vi "DEMO_HOW_TO_USE_CameraManager.vi"() -> ()   [LabVIEW 2017, in "PlayNitrideCameraComponet1010_4.lvlib"]
uses:
  <userlib>/PlayNitrideCameraComponet1010_4/PlayNitrideCameraComponet1010_4.lvlib
panel:
  out "Camera Count":i32
  out "Version":string
  out "Initial Status":bool
  out "Spend Time (ms)":u32
  out "Image":T1(plugin-control)
  in  "Camera Manager Data":T2={"Camera Index"=0.0, "Exposure Time"=2800.0, "Image"=refnum, "Save Img Path"=path "C:/Users/MyUser/Pictures", "error out"={"status"=FALSE, "code"=0, "source"=""}, "Specific Parameter"={"Parameter Name"="", "Parameter Value"=""}, "Image Info"={"Height"=0.0, "Width"=0.0, "Channels"=0.0}}
  out "Camera Manager Data Output":T2={"Camera Index"=0.0, "Exposure Time"=2800.0, "Image"=refnum, "Save Img Path"=path "C:/Users/MyUser/Pictures", "error out"={"status"=FALSE, "code"=0, "source"=""}, "Specific Parameter"={"Parameter Name"="", "Parameter Value"=""}, "Image Info"={"Height"=0.0, "Width"=0.0, "Channels"=0.0}}
  out "Commands In Queue":i32
  out "error out":errorcluster
  out "save img path":path
  in  "Pic Path":path=path "C:/Users/MyUser/Pictures/2-原圖.bmp"
  in  "Cluster In":T3={"Camera Mode"=TRUE, "顯示準星"=FALSE, "準星顏色"=65469}
  in  "Save Setting":T4
  in  "element":cluster{"State":string}
  in  "Select Command":string(combo)
  # "Select Command : 目前可以支援的指令"
  # "Initial Status : 顯示Camera Manager 是否已經成功初始化\nCamera Count: 顯示目前相機數量\n Version: 顯示目前Camera Manager dll 版號 未來用於Debug回報資訊的依據"
  # "Extra Param"
  # "Extra Output"
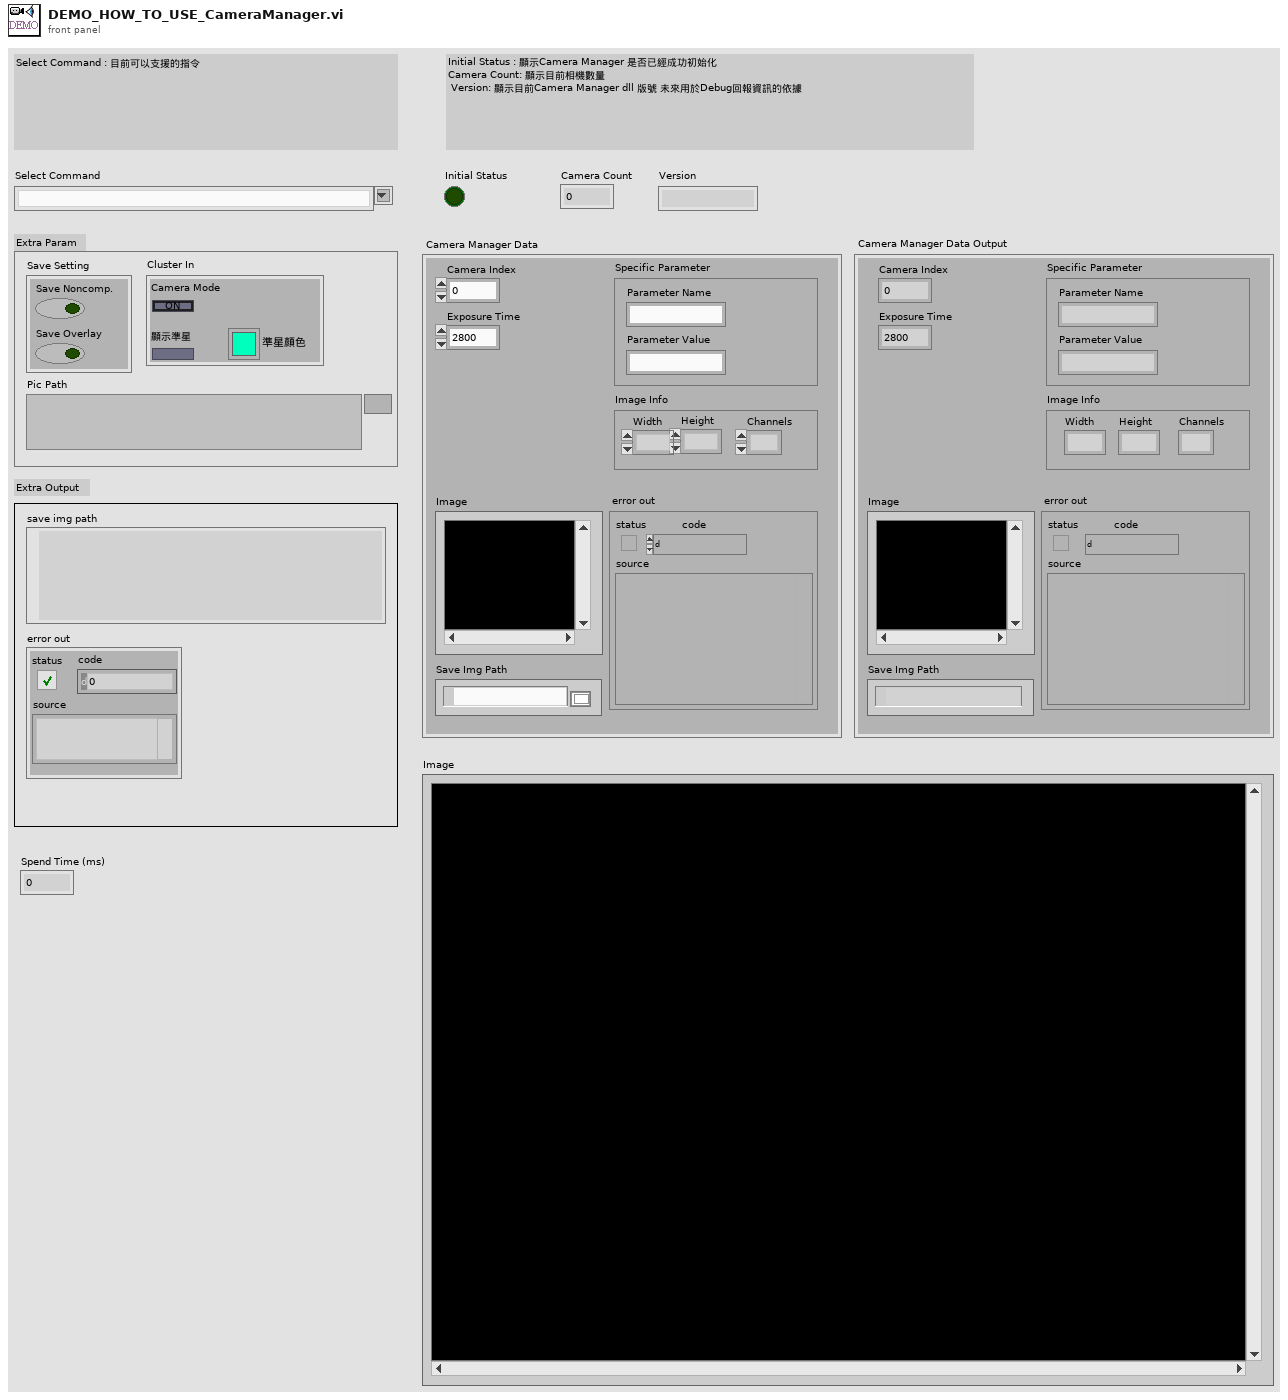
[diagram p1: front panel]
types:
  T1 = typedef "IMAQ Image.ctl" = refnum<image>
  T2 = cluster{"Camera Index":dbl, "Exposure Time":dbl, "Image":T1, "Save Img Path":path, "error out":errorcluster, "Specific Parameter":cluster{"Parameter Name":string, "Parameter Value":string}, "Image Info":cluster{"Height":dbl, "Width":dbl, "Channels":dbl}}
  T3 = cluster{"Camera Mode":bool, "顯示準星":bool, "準星顏色":u32}
  T4 = cluster{"Save Noncomp.":bool, "Save Overlay":bool}
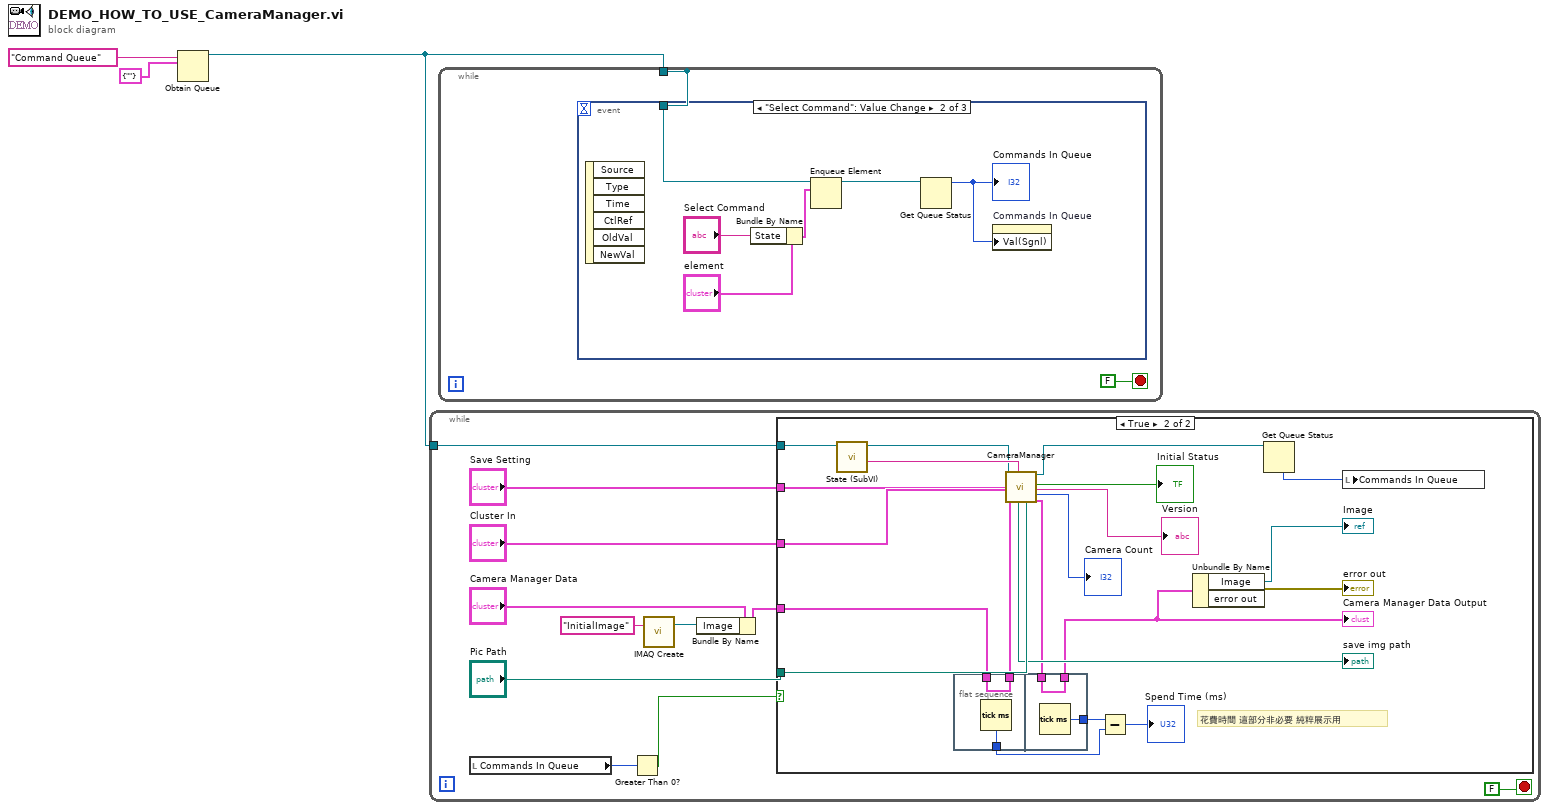
[diagram p0: block diagram]
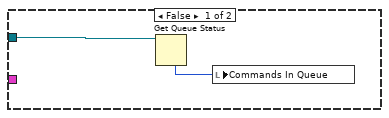
[diagram p2: hidden frame]
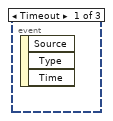
[diagram p3: hidden frame]
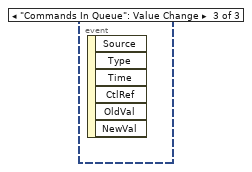
[diagram p4: hidden frame]
diagram:
  n1 = Obtain Queue(name (unnamed)="Command Queue", element data type=cluster{"State":string} {"State"=""}) -> (queue out=w1:refnum<queue>)  [unwired: 3 in, 2 out]
  n2 = while {
    tunnel: w1 -> [w11]
    stop <- FALSE stop-if-true
    n3 = local read "Commands In Queue"() -> (w14:i32)
    n4 = Greater Than 0?(x=w14) -> (x > 0?=w13:bool)
    n5 = call "IMAQ Create"("Image Name"="InitialImage") -> ("New Image"=w4:T1)  [unwired: 4 in, 1 out]
    n6 = Bundle By Name(cluster="Camera Manager Data", "Image"=w4) -> (w6:T2)
    n7 = case shown="True" w13 {
      tunnel: w11 -> [w15 w37]
      tunnel: "Save Setting" -> [_ w29]
      tunnel: "Cluster In" -> [_ w33]
      tunnel: w6 -> [_ w26]
      tunnel: "Pic Path" -> [_ w32]
      frame False {
        n8 = Get Queue Status(queue=w15) -> (# elements in queue=w16:i32)  [unwired: 2 in, 7 out]
        n9 = local write "Commands In Queue"(w16) -> ()
      }
      frame True {
        # "花費時間 這部分非必要 純粹展示用"
        n10 = call <userlib>:"State (SubVI).vi"("Queue in"=w37) -> ("State"=w36:string, "Queue out"=w35:refnum<queue>)  [unwired: 8 in, 1 out]
        n11 = flat-sequence {
          tunnel: [w39] -> w27
          tunnel: w26 -> [w39]
          tunnel: [w38] -> w23
          tunnel: [w41] -> w24
          tunnel: w25 -> [w41]
          tunnel: [w40] -> w22
          frame #0 {
            n12 = Tick Count (ms)() -> (millisecond timer value=w38:u32)
          }
          frame #1 {
            n13 = Tick Count (ms)() -> (millisecond timer value=w40:u32)
          }
        }
        n14 = call <userlib>:"CameraManager.vi"("Queue in"=w35, "Save Setting"=w29, "Cluster In"=w33, "Camera Manager Data"=w27, "Select Case"=w36, "Pic Path"=w32) -> ("save img path"=→"save img path":path, "Queue out"=w34:refnum<queue>, "Initial Status"=→"Initial Status":bool, "Version Info"=→"Version":string, "Camera Count(Output)"=→"Camera Count":i32, "Camera Manager Data Output"=w25:T2)  [unwired: 8 in]
        n15 = Subtract(x=w22, y=w23) -> (x-y=→"Spend Time (ms)":u32)
        n16 = Unbundle By Name(w24) -> ("Image"=→"Image":T1, "error out"=→"error out":errorcluster)
        n17 = Get Queue Status(queue=w34) -> (# elements in queue=w28:i32)  [unwired: 2 in, 7 out]
        n18 = local write "Commands In Queue"(w28) -> ()
        "Camera Manager Data Output" <- w24
      }
    }
  }
  n19 = while {
    tunnel: [w42] -> _
    tunnel: w1 -> [w42]
    stop <- FALSE stop-if-true
    n20 = event shown="[1] \"Select Command\": Value Change" {
      selector: _ -> [_ _ _]
      dyn-events: _ -> [_ _ _]
      timeout: _ -> [_ _ _]
      tunnel: w42 -> [_ w47 _]
      event Timeout {
        n21 = event-data() -> ()  [unwired: 1 in, 3 out]
      }
      event "Select Command": Value Change {
        n22 = event-data() -> ()  [unwired: 1 in, 6 out]
        n23 = Bundle By Name(cluster="element", "State"="Select Command") -> (w46:cluster{"State":string})
        n24 = Enqueue Element(queue=w47, element=w46) -> (queue out=w45:refnum<queue>)  [unwired: 2 in, 2 out]
        n25 = Get Queue Status(queue=w45) -> (# elements in queue=w44:i32)  [unwired: 2 in, 7 out]
        "Commands In Queue" <- w44
        n26 = property on="Commands In Queue" class="DigNum (strict)"("Val(Sgnl)"=w44) -> ()  [unwired: 2 in, 2 out]
      }
      event "Commands In Queue": Value Change {
        n27 = event-data() -> ()  [unwired: 1 in, 6 out]
      }
    }
  }
